vi "SendIntegrationControl.vi"(8 "error in (no error)":errorcluster, 10 "Integration Control Register":T1 items=["UNDEFINED"=0, "NAVX_INTEGRATION_CTL_RESET_VEL_X"=1, "NAVX_INTEGRATION_CTL_RESET_VEL_Y"=2, "NAVX_INTEGRATION_CTL_RESET_VEL_Z"=4, "NAVX_INTEGRATION_CTL_RESET_DISP_X"=8, "NAVX_INTEGRATION_CTL_RESET_DISP_Y"=16, "NAVX_INTEGRATION_CTL_RESET_DISP_Z"=32, "NAVX_INTEGRATION_CTL_RESET_YAW"=128], 11 "navX - SERIAL in":refnum<class "navX - SERIAL.lvclass">) -> (0 "error out":errorcluster, 3 "navX - SERIAL out":refnum<class "navX - SERIAL.lvclass">)   [LabVIEW 2015, in "navX Library v3.lvlib" / "navX - SERIAL.lvclass"]
uses:
  navX - SERIAL.lvclass
  navX - Interface/_TypeDefs/IntegrationControlRegisterTypeDef.ctl
  navX - SERIAL.lvclass/navX - SERIAL.ctl
  navX - Interface/navX - Interface.lvclass
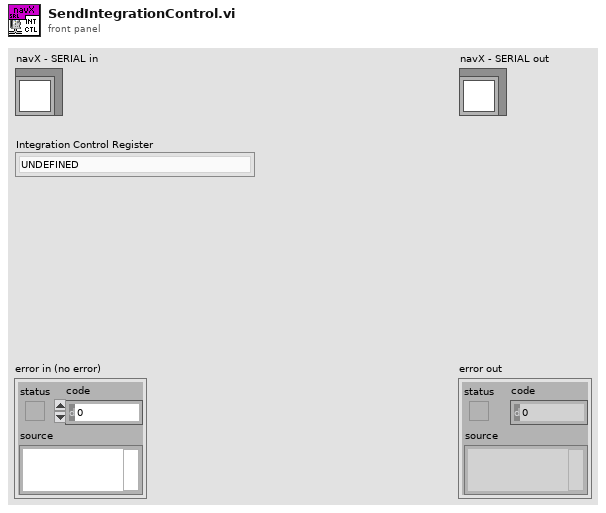
[diagram p1: front panel]
types:
  T1 = typedef "navX Library v3.lvlib/navX - Interface.lvclass/IntegrationControlRegisterTypeDef.ctl" = u8
  T2 = typedef "WPI_SerialPortRef.ctl" = cluster{"DevStatus":errorcluster, "Serial Port Name":refnum<visa-resource-name>}
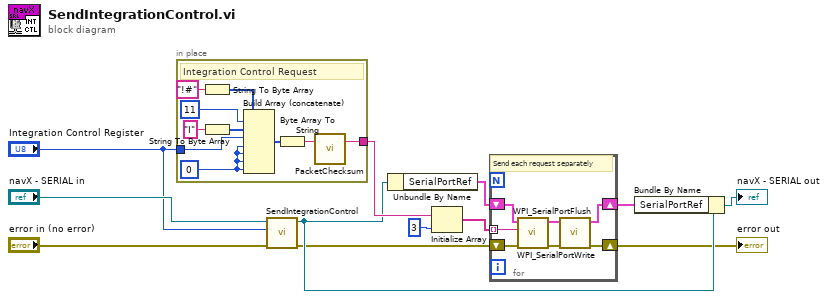
[diagram p0: block diagram]
diagram:
  n1 = in-place {
    in-place-border: [w15] -> w10
    in-place-border: "Integration Control Register" -> [w13]
    w14 = 0
    # "Integration Control Request"
    n2 = String To Byte Array(string="!#" ("initial string")) -> (unsigned byte array=w20:u8[])
    n3 = String To Byte Array(string="I" ("initial string")) -> (unsigned byte array=w18:u8[])
    n4 = Build Array (concatenate)(w20, 11, w18, w13, w14, w14, w14, w14) -> (w17:i32[])
    n5 = Byte Array To String(unsigned byte array=w17) -> (string=w16:string)
    n6 = call "PacketChecksum.vi"("Packet"=w16) -> ("Terminated Packet"=w15:string)  [unwired: 1 in, 1 out]
  }
  n7 = call-parent "SendIntegrationControl.vi"("error in (no error)"="error in (no error)", "Integration Control Register"="Integration Control Register", "navX - Interface in"="navX - SERIAL in") -> ("error out"=w4:errorcluster, "navX - Interface out"=w7:refnum<class "navX - SERIAL.lvclass">)  [unwired: 7 in]
  n8 = Unbundle By Name(w7) -> ("SerialPortRef"=w6:T2)
  n9 = Initialize Array(w10, 3 ("dimension size")) -> (w2:string[])
  n10 = for {
    tunnel: w2 -> [w27] mode=indexing
    shift-right: [w24] -> w5
    shift-left: w6 -> [w26]
    shift-right: [w23] -> w3
    shift-left: w4 -> [w25]
    # "Send each request separately"
    n11 = call <vilib>:"WPI_SerialPortWrite.vi"("error in (no error)"=w25, "Buffer"=w27, "SerialPortRef"=w26) -> ("error out"=w29:errorcluster, "SerialPortRef"=w28:T2)  [unwired: 6 in, 1 out]
    n12 = call <vilib>:"WPI_SerialPortFlush.vi"("error in (no error)"=w29, "SerialPortRef"=w28) -> ("error out"=w23:errorcluster, "SerialPortRef"=w24:T2)  [unwired: 8 in]
  }
  "error out" <- w3
  n13 = Bundle By Name(cluster=w7, "SerialPortRef"=w5) -> (→"navX - SERIAL out":refnum<class "navX - SERIAL.lvclass">)
